vi "Uebersicht Ausgabefelder einfaerben.vi"(6 "Aktionen":T1, 11 "Angehängtes Array":refnum<vi>[](array[refnum])) -> ()   [LabVIEW 2020, in "Anlagenuebersicht.lvlib"]
uses:
  VisBx Anzeige/Anlagenuebersicht.lvlib
  Aktionen Ausgabefaelder einfaerben.ctl
  Anlagengrenzwerte/FGV Anlagengrenzwerte Aktionen.ctl
  Anlagengrenzwerte/Anlagen-Parameter Anzeige.ctl
  Funktionstasten/Funktionstasten-Aktion.ctl
  Funktionstasten/Zustaende.ctl
  Allgemein/allgemeine Sub-VIs.lvlib
  Anlagengrenzwerte/Anlagengrenzwerte.lvlib
  Funktionstasten/Funktionstasten.lvlib
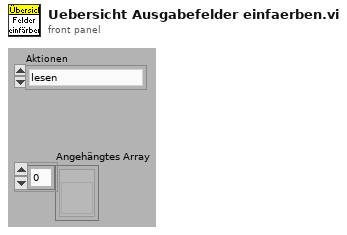
[diagram p1: front panel]
types:
  T1 = typedef "Anlagenuebersicht.lvlib/Aktionen Ausgabefaelder einfaerben.ctl" = enum16{"lesen", "prüfen", "initialisieren"}
  T2 = typedef "Funktionstasten.lvlib/Zustaende.ctl" = enum16{"Standby", "Pause", "Eco", "Messen", "Kalibrieren", "Spülen Filter", "Spülen Leitung", "Umgebungsluft", "0-Gas", "Cal-Gas", "CG zu PNS", "-------------", "Init 1", "Init 2", "Init 3", "Init 4", "Messen vorbereiten", "Messen durchführen", "Exit"}
  T3 = typedef "Funktionstasten.lvlib/Funktionstasten-Aktion.ctl" = enum16{"Initialisieren", "Zustand setzen", "Taste gedrückt", "Fehler speichern", "Lesen", "Manuell", "Remote", "Bitparallel", "Samplepoint", "Zeit Prüfen", "reset Umschalten"}
  T4 = typedef "Anlagengrenzwerte.lvlib/Anlagen-Parameter Anzeige.ctl" = cluster{"Sollwert":sgl, "Warn-Min":sgl, "Warn-Max":sgl, "Abschalt-Min":sgl, "Abschalt-Max":sgl, "Regler":u16}
  T5 = typedef "Anlagengrenzwerte.lvlib/FGV Anlagengrenzwerte Aktionen.ctl" = enum16{"Lesen", "Grenzwerte schreiben"}
  T6 = typedef "Anlagengrenzwerte.lvlib/Anlagen-Grenzwerte Anzeige.ctl" = cluster{"Eingangsdruck FT-IR:":T4, "Durchfluss FT-IR:":T4, "Durchfluss CalGas:":T4, "Druck Ausgang:":T4, "Druck Kalter Block:":T4, "Heizleitungen intern:":T4, "Heizleitung zu FT-IR:":T4, "Heizung Filterblock:":T4, "Heizung Pumpe:":T4, "Heizleitung Extern SP1:":T4, "Heizleitung Extern SP2:":T4, "FT-IR Heizung Messzelle:":T4, "Schaltschranktemperatur:":T4, "Gaskühler:":T4}
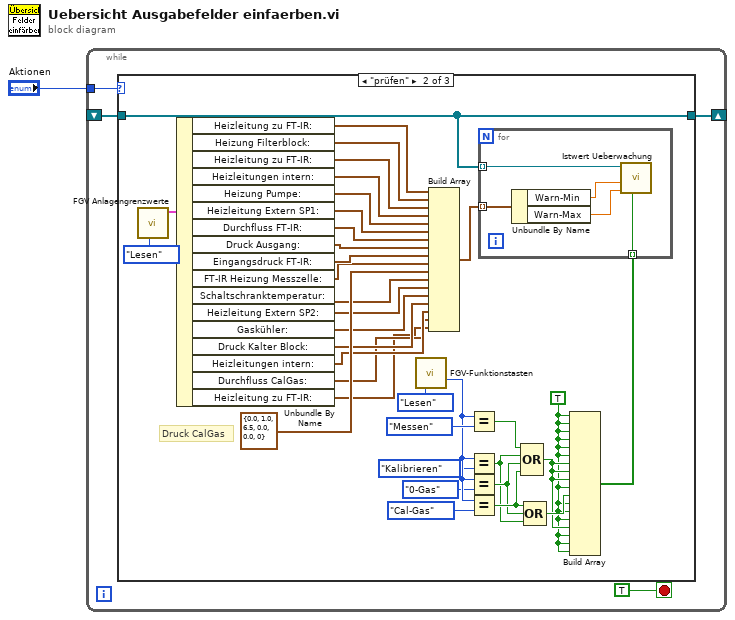
[diagram p0: block diagram]
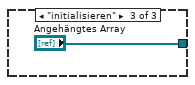
[diagram p3: hidden frame]
diagram:
  n1 = while {
    tunnel: "Aktionen" -> [w5]
    shift-right: [w4] -> _
    shift-left: _ -> [w3]
    stop <- TRUE stop-if-true
    n2 = case shown="\"prüfen\"" w5 {
      tunnel: [w6 w33 "Angehängtes Array"] -> w4
      tunnel: w3 -> [w6 w33 _]
      frame "lesen", Default {
      }
      frame "prüfen" {
        w7 = TRUE
        # "Druck CalGas"
        n3 = call "FGV Anlagengrenzwerte.vi"("Aktion"=FGV_Anlagengrenzwerte_Aktionen."Lesen") -> ("Anlagen-Grenzwerte Anzeige"=w31:T6)  [unwired: 10 in]
        n4 = Unbundle By Name(w31) -> ("Heizleitung zu FT-IR:"=w10:T4, "Heizung Filterblock:"=w42:T4, "Heizleitung zu FT-IR:"=w41:T4, "Heizleitungen intern:"=w40:T4, "Heizung Pumpe:"=w39:T4, "Heizleitung Extern SP1:"=w38:T4, "Durchfluss FT-IR:"=w37:T4, "Druck Ausgang:"=w36:T4, "Eingangsdruck FT-IR:"=w35:T4, "FT-IR Heizung Messzelle:"=w30:T4, "Schaltschranktemperatur:"=w16:T4, "Heizleitung Extern SP2:"=w15:T4, "Gaskühler:"=w14:T4, "Druck Kalter Block:"=w13:T4, "Heizleitungen intern:"=w11:T4, "Durchfluss CalGas:"=w9:T4, "Heizleitung zu FT-IR:"=w8:T4)
        n5 = call "FGV-Funktionstasten.vi"("Aktion"=Funktionstasten-Aktion."Lesen") -> ("ausgewählte Funktion"=w25:T2)  [unwired: 7 in, 7 out]
        n6 = Build Array(w10, w42, w41, w40, w39, w38, w37, w36, w35, w30, T4 {"Sollwert"=0.0, "Warn-Min"=1.0, "Warn-Max"=6.5, "Abschalt-Min"=0.0, "Abschalt-Max"=0.0, "Regler"=0} ("Element"), w16, w15, w14, w13, w11, w9, w8) -> (w34:T4[])
        n7 = Equal?(x=w25, y=Zustaende."Messen") -> (x = y?=w27:bool)
        n8 = Equal?(x=w25, y=Zustaende."Kalibrieren") -> (x = y?=w19:bool)
        n9 = Equal?(x=w25, y=Zustaende."0-Gas") -> (x = y?=w20:bool)
        n10 = Equal?(x=w25, y=Zustaende."Cal-Gas") -> (x = y?=w21:bool)
        n11 = Compound Arithmetic op=OR(w27, w19, w20, w21) -> (w12:bool)
        n12 = Compound Arithmetic op=OR(w21, w20, w19) -> (w18:bool)
        n13 = Build Array(w7, w7, w7, w7, w7, w7, w12, w12, w12, w7, w18, w7, w7, w7, w12, w7, w7, w7) -> (w17:bool[])
        n14 = for {
          tunnel: w33 -> [w44] mode=indexing
          tunnel: w34 -> [w47] mode=indexing
          tunnel: w17 -> [w43] mode=indexing
          n15 = Unbundle By Name(w47) -> ("Warn-Min"=w46:sgl, "Warn-Max"=w45:sgl)
          n16 = call "Istwert Ueberwachung.vi"("Fehler Aktiviert?"=w43, "Max"=w45, "Min"=w46, "Referernz"=w44) -> ()  [unwired: 8 in]
        }
      }
      frame "initialisieren" {
      }
    }
  }
